vi "Start Count Down.vi"(8 "error in (no error)":errorcluster, 10 "Seconds To Wait":i32, 11 "Timer Actor in":refnum<class "Timer Actor.lvclass">) -> (0 "error out":errorcluster, 3 "Timer Actor out":refnum<class "Timer Actor.lvclass">)   [LabVIEW 2024, in "Timer Actor.lvlib" / "Timer Actor.lvclass"]
uses:
  Timer Actor.lvclass
  Timer Actor Messages/Send Count Down Finished Msg/Send Count Down Finished Msg.lvclass
  <vilib>/ActorFramework/Actor/Actor.lvclass/Actor.ctl
  <vilib>/ActorFramework/Message Enqueuer/Message Enqueuer.lvclass/Message Enqueuer.ctl
  Timer Actor.lvclass/Timer Actor.ctl
  <vilib>/ActorFramework/Message Enqueuer/Init from Existing Queue.vi
  <vilib>/ActorFramework/Message Enqueuer/Message Enqueuer.lvclass
  <vilib>/ActorFramework/Actor/Actor.lvclass
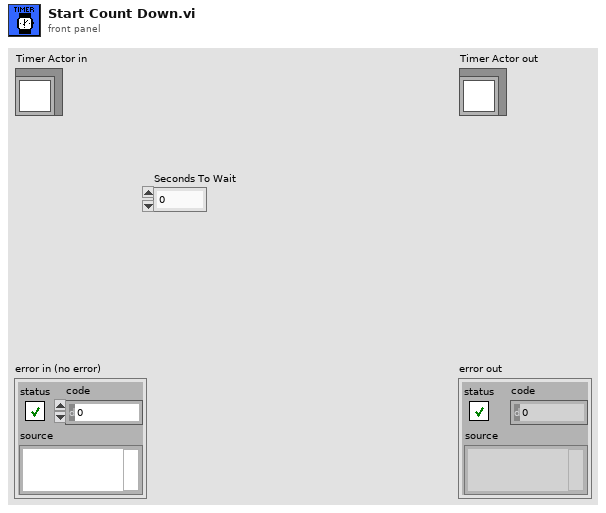
[diagram p1: front panel]
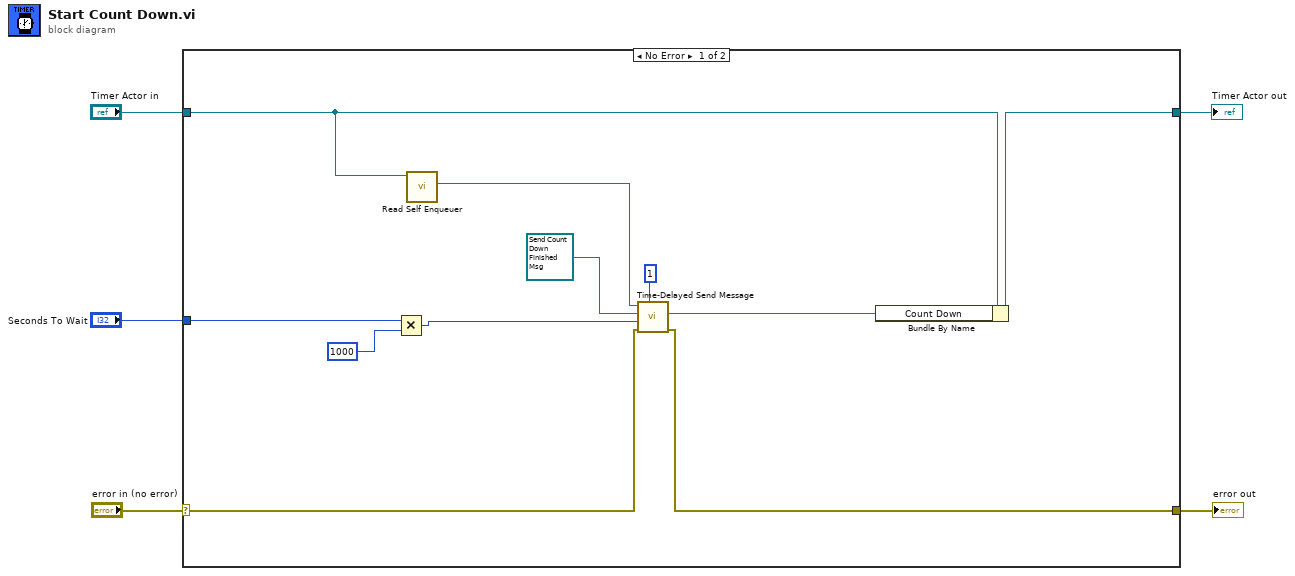
[diagram p0: block diagram]
diagram:
  n1 = case shown="No Error" "error in (no error)" {
    selector: "error in (no error)" -> [w16 w18]
    tunnel: [w15 w18] -> w4
    tunnel: [w7 w17] -> w2
    tunnel: "Timer Actor in" -> [w13 w17]
    tunnel: "Seconds To Wait" -> [w10 _]
    frame No Error {
      n2 = Multiply(x=w10, y=1000) -> (x*y=w9:i32)
      n3 = call <vilib>:"Read Self Enqueuer.vi"("Actor"=w13) -> ("Self Enqueuer"=w14:refnum<class "Message Enqueuer.lvclass">)  [unwired: 10 in]
      n4 = call <vilib>:"Time-Delayed Send Message.vi"("# Copies (0 = infinite repeat)"=u32 1, "error in (no error)"=w16, "Milliseconds To Wait"=w9, "Message"=refnum<class "Send Count Down Finished Msg.lvclass"> refnum ("Timer Actor.lvlib:Send Count Down Finished Msg.lvclass"), "Message Enqueuer"=w14) -> ("error out"=w15:errorcluster, "Delivery Notifier"=w6:refnum<notifier>)  [unwired: 5 in]
      n5 = Bundle By Name(cluster=w13, "Count Down"=w6) -> (w7:refnum<class "Timer Actor.lvclass">)
    }
    frame Error {
    }
  }
  "error out" <- w4
  "Timer Actor out" <- w2
